vi "Isotopic Centrifuge.vi"(4 "Speed Upgrades":u32 max=8, 7 "Uranium Hexaflouride (mB/t)":ext) -> (0 "Input Limiting":bool, 1 "Limiting":bool, 3 "Fissile Fuel (mB/t)":ext format="%.2f")   [LabVIEW 2023]
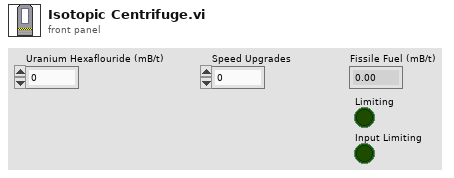
[diagram p1: front panel]
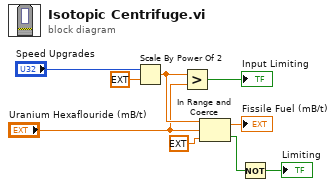
[diagram p0: block diagram]
diagram:
  n1 = Scale By Power Of 2(n="Speed Upgrades", x=ext 1.0) -> (x*2^n=w3:ext)
  n2 = Greater?(x=w3, y="Uranium Hexaflouride (mB/t)") -> (0:→"Input Limiting":bool)
  n3 = In Range and Coerce(upper limit=w3, x="Uranium Hexaflouride (mB/t)", lower limit=ext 0.0) -> (coerced(x)=→"Fissile Fuel (mB/t)":ext, In Range?=w5:bool)
  n4 = Not(x=w5) -> (.not. x?=→"Limiting":bool)
